vi "TrackingComm.vi"(2 "OWL Freq Hz(default: 480)":dbl=480.0 format="%.1f", 3 "marker tally (default: 32)":i32=32, 4 "server address":string="192.168.0.101") -> (0 "error out":errorcluster, 1 "connected to server?":bool)   [LabVIEW 2011]
uses:
  ctrInitFlags.ctl
  ctrCommonFlags.ctl
  ctrTrackersFlags.ctl
  ctrMarkersFlags.ctl
  ctrSetsFlags.ctl
  C:/Program Files/Phasespace/libowlsock.dll
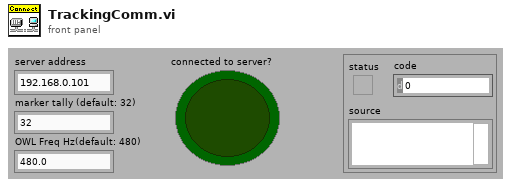
[diagram p1: front panel]
types:
  T1 = typedef "ctrInitFlags.ctl" = u16
  T2 = typedef "ctrCommonFlags.ctl" = u16
  T3 = typedef "ctrTrackersFlags.ctl" = u16
  T4 = typedef "ctrMarkersFlags.ctl" = u16
  T5 = typedef "ctrSetsFlags.ctl" = u16
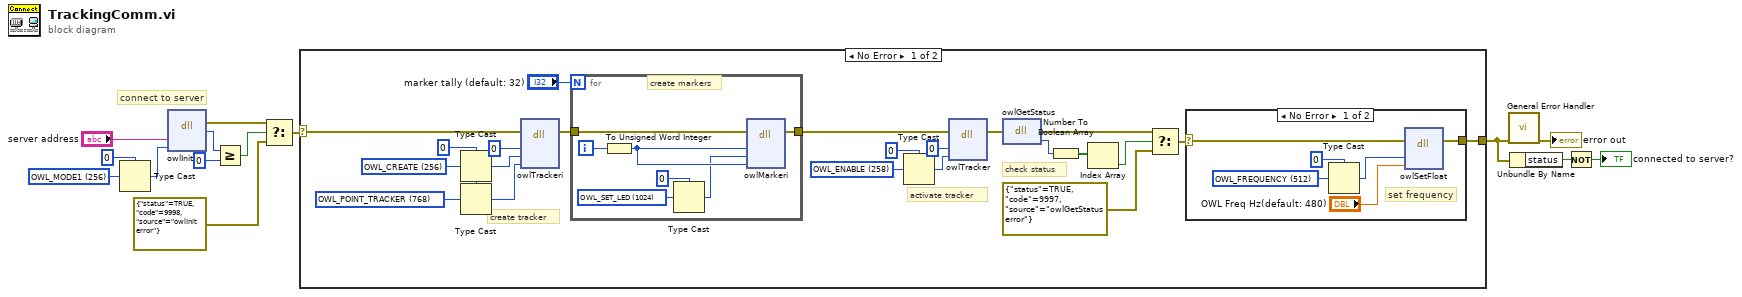
[diagram p0: block diagram]
diagram:
  w3 = T1 256 items=["OWL_SLAVE"=1, "OWL_FILE"=2, "OWL_POSTPROCESS"=16, "OWL_MODE1"=256, "OWL_MODE2"=512, "OWL_MODE3"=768, "OWL_MODE4"=1024, "OWL_LASER"=2560, "OWL_CALIB"=3072, "OWL_CALIBPLANAR"=3840]
  # "connect to server"
  n1 = Type Cast(type=u16 0, x=w3) -> (*(type *) &x=w2:u16)
  n2 = dll-call lib="C:/Program Files/Phasespace/libowlsock.dll" fn="owlInit"("server"="server address", "flags"=w2) -> (error out=w9:errorcluster, "return type"=w13:i16)  [unwired: 5 in, 1 out]
  n3 = Greater Or Equal?(x=w13, y=i16 0) -> (x >= y?=w10:bool)
  n4 = Select(t=w9, s=w10, f=errorcluster {"status"=TRUE, "code"=9998, "source"="owlInit error"} ("error out")) -> (s? t:f=w8:errorcluster)
  n5 = case shown="No Error" w8 {
    selector: w8 -> [w35 w51]
    tunnel: [w36 w51] -> w6
    frame No Error {
      w19 = T2 258 items=["OWL_CREATE"=256, "OWL_DESTROY"=257, "OWL_ENABLE"=258, "OWL_DISABLE"=259] ("Common flages")
      w22 = T3 768 items=["OWL_POINT_TRACKER"=768, "OWL_RIGID_TRACKER"=769]
      w21 = u16 0 ("y")
      w25 = T2 256 items=["OWL_CREATE"=256, "OWL_DESTROY"=257, "OWL_ENABLE"=258, "OWL_DISABLE"=259] ("Common flages")
      # "activate tracker"
      # "create tracker"
      # "check status"
      n6 = Type Cast(type=w21, x=w25) -> (*(type *) &x=w24:u16)
      n7 = Type Cast(type=w21, x=w22) -> (*(type *) &x=w23:u16)
      n8 = dll-call lib="C:/Program Files/Phasespace/libowlsock.dll" fn="owlTrackeri"(error in=w35, "tracker"=u16 0 ("y"), "pname"=w24, "param"=w23) -> (error out=w31:errorcluster)  [unwired: 5 in, 2 out]
      n9 = for {
        N: "marker tally (default: 32)" -> [_]
        tunnel: w31 -> [w42]
        tunnel: [w41] -> w32
        i -> [w43]
        w39 = T4 1024 items=["OWL_SET_LED"=1024, "OWL_SET_POSITION"=1025, "OWL_CLEAR_MARKER"=1026]
        # "create markers"
        n10 = To Unsigned Word Integer(number=w43) -> (unsigned 16bit integer=w40:u16)
        n11 = Type Cast(type=u16 0 ("y"), x=w39) -> (*(type *) &x=w38:u16)
        n12 = dll-call lib="C:/Program Files/Phasespace/libowlsock.dll" fn="owlMarkeri"(error in=w42, "marker"=w40, "pname"=w38, "param"=w40) -> (error out=w41:errorcluster)  [unwired: 5 in, 2 out]
      }
      n13 = Type Cast(type=u16 0 ("y"), x=w19) -> (*(type *) &x=w18:u16)
      n14 = dll-call lib="C:/Program Files/Phasespace/libowlsock.dll" fn="owlTracker"(error in=w32, "tracker"=u16 0, "pname"=w18) -> (error out=w34:errorcluster)  [unwired: 4 in, 2 out]
      n15 = dll-call lib="C:/Program Files/Phasespace/libowlsock.dll" fn="owlGetStatus"(error in=w34) -> (error out=w28:errorcluster, "return type"=w17:u16)  [unwired: 2 in, 1 out]
      n16 = Number To Boolean Array(number=w17) -> (Boolean array=w16:bool[])
      n17 = Index Array(array=w16) -> (element=w15:bool)  [unwired: 1 in]
      n18 = Select(t=w28, s=w15, f=errorcluster {"status"=TRUE, "code"=9997, "source"="owlGetStatus error"} ("error out")) -> (s? t:f=w27:errorcluster)
      n19 = case shown="No Error" w27 {
        selector: w27 -> [w49 w50]
        tunnel: [w48 w50] -> w36
        frame No Error {
          w45 = T5 512 items=["OWL_FREQUENCY"=512, "OWL_STREAMING"=513, "OWL_INTERPOLATION"=514, "OWL_BUTTONS"=528, "OWL_MARKERS"=529, "OWL_RIGIDS"=530, "OWL_COMMDATA"=544, "OWL_TIMESTAMP"=545, "OWL_PLANES"=672, "OWL_DETECTORS"=673, "OWL_IMAGES"=674, "OWL_TRANSFORM"=49664]
          # "set frequency"
          n20 = Type Cast(type=u16 0 ("y"), x=w45) -> (*(type *) &x=w46:u16)
          n21 = dll-call lib="C:/Program Files/Phasespace/libowlsock.dll" fn="owlSetFloat"(error in=w49, "pname"=w46, "param"="OWL Freq Hz(default: 480)") -> (error out=w48:errorcluster)  [unwired: 4 in, 2 out]
        }
        frame Error {
        }
      }
    }
    frame Error {
    }
  }
  n22 = call <vilib>:"General Error Handler.vi"("error in (no error)"=w6) -> ("error out"=→"error out":errorcluster)  [unwired: 2 in, 12 out]
  n23 = Unbundle By Name(w6) -> ("status"=w5:bool)
  n24 = Not(x=w5) -> (.not. x?=→"connected to server?":bool)
